vi "Read Vertical Scrollbar.vi"(9 "String in":refnum<class "String.lvclass">) -> (3 "String out":refnum<class "String.lvclass">, 4 "Vertical Scrollbar":bool)   [LabVIEW 2014, in "String.lvclass"]
uses:
  String.lvclass
  String.lvclass/String.ctl
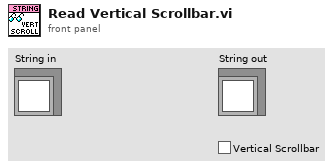
[diagram p1: front panel]
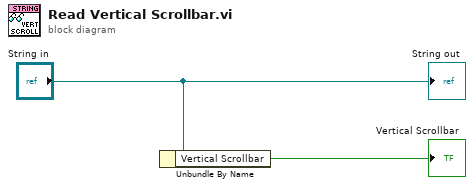
[diagram p0: block diagram]
diagram:
  n1 = Unbundle By Name("String in") -> ("Vertical Scrollbar"=→"Vertical Scrollbar":bool)
  "String out" <- "String in"
